vi "PH_ImageStatistician.panel.vi"(0 "object ref":refnum<vi>, 5 "error in (no error)":errorcluster) -> (19 "error out":errorcluster)   [LabVIEW 2014, in "PH_ImageStatistician.lvlib"]
doc: "This is just an example for a GUI thread.\n\nLicense Agreement for this software:\n\nCopyright (C)\nGesellschaft für Schwerionenforschung, GSI\nPlanckstr. 1\n64291 Darmstadt\nGermany\n\nContact: D.Beck@gsi.de \n\nThis program is free software; you can redistribute it and/or modify it under the terms of the GNU General Public License as published by the Free Software Foundation; either version 2 of the license, or (at your option) any later version.\n\nThis program is distributed in the hope that it will be useful, but WITHOUT ANYW ARRANTY; without even the implied warranty of MERCHANTABILITY or FITNESS FOR A PARTICULAR PURPOSE. See the GNU General License for more details (http://www.gnu.org).\n\nGesellschaft für Schwerionenforschung, GSI\nPlanckstr. 1, 64291 Darmstadt, Germany\nFor all questions and ideas contact: M.Richter@gsi.de, H.Brand@gsi.de or D.Beck@gsi.de.\nLast update: 18-DEC-2002"
uses:
  PH_ImageStatistician.lvlib
  PH_ImageStatistician.select Data.ctl
  PH_Common/PH_Common.lvlib
  CSCore/CSSystem/CSSystemLib/CSSystemLib.lvlib
  PH_Class/PH_Class.lvlib
panel:
  in  "Start":bool
  in  "Stat or Trend":bool
  in  "Export Data":bool
  out "Result Graph":cluster{dbl[], dbl[]}[](graph)
  out "Std Dev Data 3":dbl caption="Unit" format="%#_4g"
  in  "Dummy Std Dev":string caption="Std Dev"
  in  "Dummy Mean":string caption="Mean"
  out "Mean Data 3":dbl caption="Unit" format="%#_4g"
  out "Std Dev Data 2":dbl caption="Unit" format="%#_4g"
  out "Mean Data 2":dbl caption="Unit" format="%#_4g"
  out "Std Dev Data 1":dbl caption="Unit" format="%#_4g"
  out "Mean Data 1":dbl caption="Unit" format="%#_4g"
  in  "Data 3":T1 items=["nothing ", "FWHM Major Trace", "FWHM Minor Trace", "Gaussian Fit Order Major Trace", "Gaussian Fit Order Minor Trace", "99% Diameter Major Trace", "99% Diameter Minor Trace", "Theta", "Delta", "Major Diameter", "Minor Diameter", "Azimuth Angle", "Azi Angle rel to Major?", "Ellipticity", "Center of gravity - x", "Center of gravity - y", "Energy"]
  in  "Data 2":T1 items=["nothing ", "FWHM Major Trace", "FWHM Minor Trace", "Gaussian Fit Order Major Trace", "Gaussian Fit Order Minor Trace", "99% Diameter Major Trace", "99% Diameter Minor Trace", "Theta", "Delta", "Major Diameter", "Minor Diameter", "Azimuth Angle", "Azi Angle rel to Major?", "Ellipticity", "Center of gravity - x", "Center of gravity - y", "Energy"]
  in  "Data 1":T1 items=["nothing ", "FWHM Major Trace", "FWHM Minor Trace", "Gaussian Fit Order Major Trace", "Gaussian Fit Order Minor Trace", "99% Diameter Major Trace", "99% Diameter Minor Trace", "Theta", "Delta", "Major Diameter", "Minor Diameter", "Azimuth Angle", "Azi Angle rel to Major?", "Ellipticity", "Center of gravity - x", "Center of gravity - y", "Energy"]
  out "Status":u32(colorbox)
  in  "Operator":string
  in  "Delete":bool
  # "PCS"
  # "3.40"
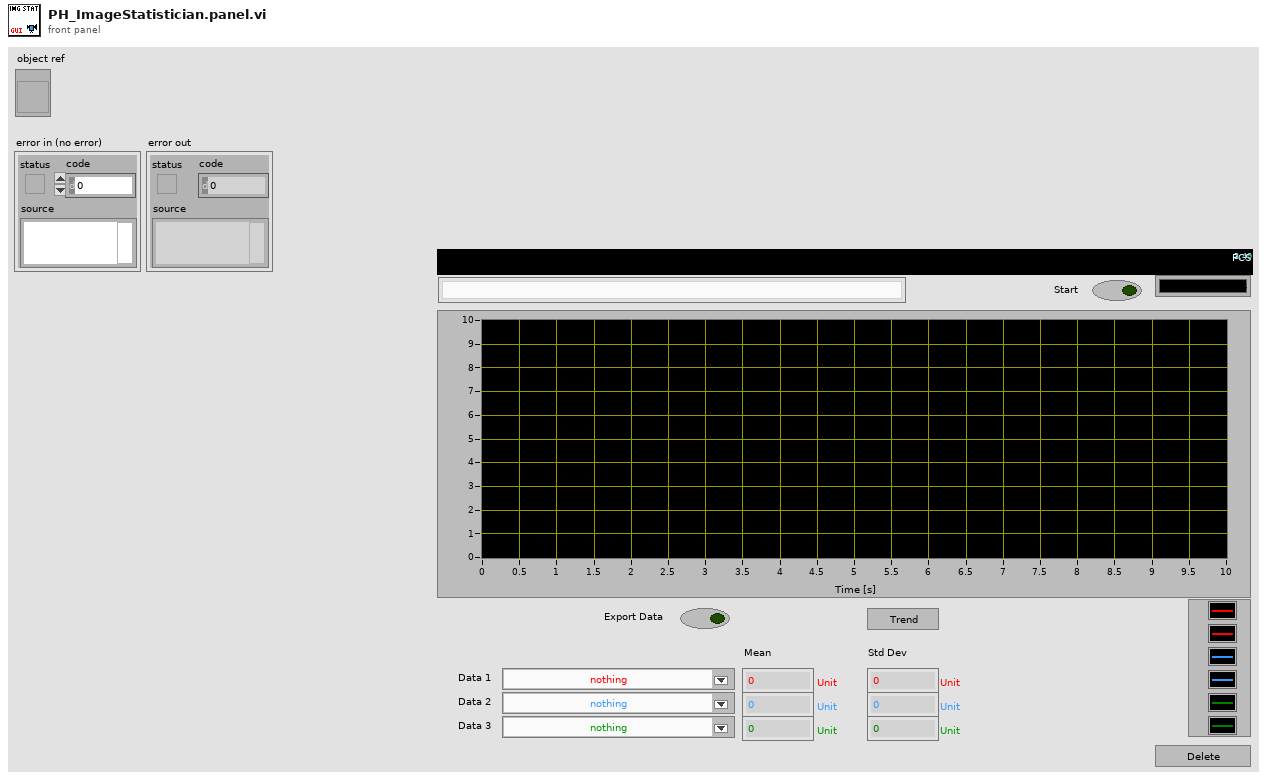
[diagram p1: front panel]
types:
  T1 = typedef "PH_ImageStatistician.lvlib/PH_ImageStatistician.select Data.ctl" = u16
  T2 = enum8{"Enabled", "Disabled", "Disabled and Grayed Out"}
  T3 = typedef "PH_ImageStatistician.lvlib/PH_ImageStatistician.i attribute.ctl" = cluster{"GUI Refs ":cluster{"Status":refnum<vi>, "Result Graph":refnum<vi>, "Mean Data 1":refnum<vi>, "Std Dev Data 1":refnum<vi>, "Mean Data 2":refnum<vi>, "Std Dev Data 2":refnum<vi>, "Mean Data 3":refnum<vi>, "Std Dev Data 3":refnum<vi>, "Dummy Mean":refnum<vi>, "Dummy Std Dev":refnum<vi>, "Export Data":refnum<vi>, "Data 1":refnum<vi>, "Data 2":refnum<vi>, "Data 3":refnum<vi>, "Stat or Trend":refnum<vi>, "Delete":refnum<vi>, "Operator":refnum<vi>, "Start":refnum<vi>}, "Operator":string, "Data":T4[], "Stat or Trend":bool, "Data 1":T1, "Data 2":T1, "Data 3":T1, "Start":bool, "Datasets strored":i32, "Dataarray Size":i32}
  T4 = typedef "PH_ImageStatistician.lvlib/PH_ImageStatistician.Statistician Data.ctl" = cluster{"Snapshot Time":dbl, "Maj FWHM":dbl, "Min FWHM":dbl, "Maj Fit Order":dbl, "Min Fit Order":dbl, "99% Diam Maj Trace":dbl, "99% Diam Min Trace":dbl, "Theta":dbl, "Delta":dbl, "Maj Diam":dbl, "Min Diam":dbl, "Azimuth Angle":dbl, "Azi Angle rel to major?":dbl, "Ellipticity":dbl, "CoG - X":dbl, "CoG - Y":dbl, "Energy":dbl, "Energy Cal - no mJ":dbl, "Lin Cal - no mm or mrad":dbl, "Lin Cal Factor":dbl}
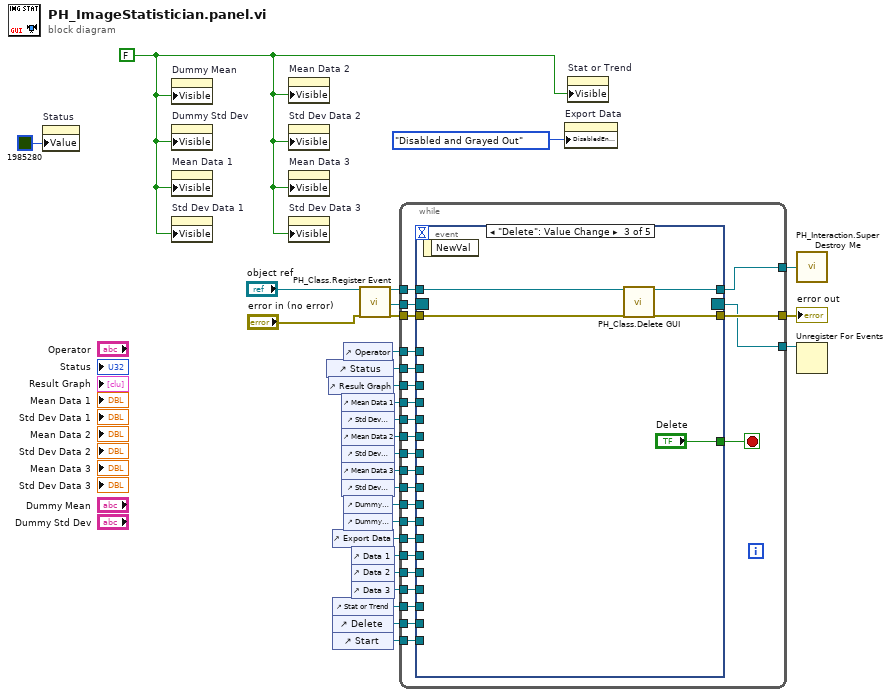
[diagram p0: block diagram]
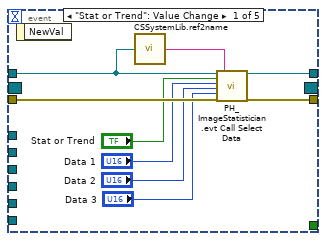
[diagram p2: hidden frame]
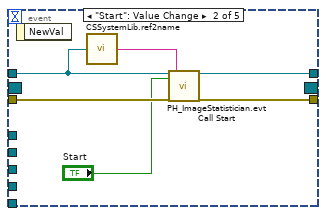
[diagram p3: hidden frame]
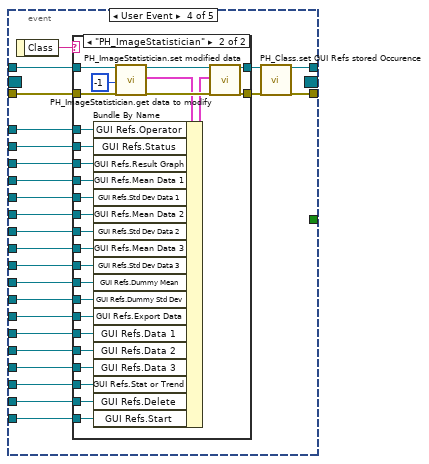
[diagram p4: hidden frame]
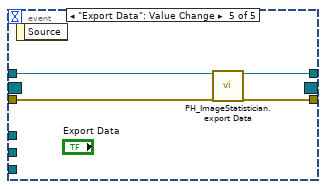
[diagram p6: hidden frame]
diagram:
  w27 = FALSE
  n1 = property on="Status" class="ColBox"("Value"=u32 1985280 ("Status")) -> ()  [unwired: 2 in, 2 out]
  n2 = property on="Dummy Mean" class="Str"("Visible"=w27) -> ()  [unwired: 2 in, 2 out]
  n3 = property on="Dummy Std Dev" class="Str"("Visible"=w27) -> ()  [unwired: 2 in, 2 out]
  n4 = property on="Mean Data 1" class="DigNum (strict)"("Visible"=w27) -> ()  [unwired: 2 in, 2 out]
  n5 = property on="Std Dev Data 1" class="DigNum (strict)"("Visible"=w27) -> ()  [unwired: 2 in, 2 out]
  n6 = property on="Mean Data 2" class="DigNum (strict)"("Visible"=w27) -> ()  [unwired: 2 in, 2 out]
  n7 = property on="Std Dev Data 2" class="DigNum (strict)"("Visible"=w27) -> ()  [unwired: 2 in, 2 out]
  n8 = property on="Mean Data 3" class="DigNum (strict)"("Visible"=w27) -> ()  [unwired: 2 in, 2 out]
  n9 = property on="Std Dev Data 3" class="DigNum (strict)"("Visible"=w27) -> ()  [unwired: 2 in, 2 out]
  n10 = control-ref of="Status"() -> (w17:refnum<vi>)
  n11 = control-ref of="Result Graph"() -> (w16:refnum<vi>)
  n12 = control-ref of="Export Data"() -> (w7:refnum<vi>)
  n13 = control-ref of="Stat or Trend"() -> (w3:refnum<vi>)
  n14 = control-ref of="Delete"() -> (w2:refnum<vi>)
  n15 = control-ref of="Start"() -> (w1:refnum<vi>)
  n16 = control-ref of="Mean Data 1"() -> (w15:refnum<vi>)
  n17 = control-ref of="Std Dev Data 1"() -> (w14:refnum<vi>)
  n18 = control-ref of="Mean Data 2"() -> (w13:refnum<vi>)
  n19 = control-ref of="Std Dev Data 2"() -> (w12:refnum<vi>)
  n20 = control-ref of="Mean Data 3"() -> (w11:refnum<vi>)
  n21 = control-ref of="Std Dev Data 3"() -> (w10:refnum<vi>)
  n22 = control-ref of="Operator"() -> (w18:refnum<vi>)
  n23 = control-ref of="Dummy Mean"() -> (w9:refnum<vi>)
  n24 = control-ref of="Dummy Std Dev"() -> (w8:refnum<vi>)
  n25 = control-ref of="Data 1"() -> (w6:refnum<vi>)
  n26 = control-ref of="Data 2"() -> (w5:refnum<vi>)
  n27 = control-ref of="Data 3"() -> (w4:refnum<vi>)
  n28 = call "PH_Class.Register Event.vi"("i ref in"="object ref", "error in (no error)"="error in (no error)") -> ("i ref out"=w24:refnum<vi>, "Event Registration Refnum"=w22:refnum<event-registration>, "error out"=w23:errorcluster)  [unwired: 15 in]
  n29 = while {
    tunnel: w24 -> [w53]
    tunnel: [w52] -> w29
    tunnel: [w51] -> w28
    tunnel: w23 -> [w50]
    tunnel: w22 -> [w49]
    tunnel: [w48] -> w21
    tunnel: w18 -> [w47]
    tunnel: w17 -> [w46]
    tunnel: w16 -> [w45]
    tunnel: w15 -> [w44]
    tunnel: w14 -> [w43]
    tunnel: w13 -> [w42]
    tunnel: w12 -> [w41]
    tunnel: w11 -> [w40]
    tunnel: w10 -> [w39]
    tunnel: w9 -> [w38]
    tunnel: w8 -> [w37]
    tunnel: w7 -> [w36]
    tunnel: w6 -> [w35]
    tunnel: w5 -> [w34]
    tunnel: w4 -> [w33]
    tunnel: w3 -> [w32]
    tunnel: w2 -> [w31]
    tunnel: w1 -> [w30]
    stop <- w54 stop-if-true
    n30 = event shown="[2] \"Delete\": Value Change" {
      selector: w49 -> [_ _ _ _ _]
      dyn-events: [_ _ _ _ _] -> w48
      timeout: _ -> [_ _ _ _ _]
      tunnel: [_ _ "Delete" _ _] -> w54
      tunnel: w53 -> [w59 w65 w73 w99 w131]
      tunnel: [w61 w67 w72 w95 w129] -> w52
      tunnel: [w62 w68 w70 w94 w130] -> w51
      tunnel: w50 -> [w63 w69 w71 w98 w132]
      tunnel: w47 -> [_ _ _ w92 _]
      tunnel: w46 -> [_ _ _ w91 _]
      tunnel: w45 -> [_ _ _ w90 _]
      tunnel: w44 -> [_ _ _ w89 _]
      tunnel: w43 -> [_ _ _ w88 _]
      tunnel: w42 -> [_ _ _ w87 _]
      tunnel: w41 -> [_ _ _ w86 _]
      tunnel: w40 -> [_ _ _ w85 _]
      tunnel: w39 -> [_ _ _ w84 _]
      tunnel: w38 -> [_ _ _ w83 _]
      tunnel: w37 -> [_ _ _ w82 _]
      tunnel: w36 -> [_ _ _ w81 _]
      tunnel: w35 -> [_ _ _ w80 _]
      tunnel: w34 -> [_ _ _ w79 _]
      tunnel: w33 -> [_ _ _ w78 _]
      tunnel: w32 -> [_ _ _ w77 _]
      tunnel: w31 -> [_ _ _ w76 _]
      tunnel: w30 -> [_ _ _ w75 _]
      event "Stat or Trend": Value Change {
        n31 = event-data() -> ()  [unwired: 1 in, 1 out]
        n32 = call "CSSystemLib.ref2name.vi"("obj refnum"=w59) -> ("name"=w60:string)
        n33 = call "PH_ImageStatistician.evt Call Select Data.vi"("i ref in"=w59, "Stat or Trend"="Stat or Trend", "Data 1"="Data 1", "Data 2"="Data 2", "Data 3"="Data 3", "error in (no error)"=w63, "Instance"=w60) -> ("i ref out"=w61:refnum<vi>, "error out"=w62:errorcluster)  [unwired: 11 in]
      }
      event "Start": Value Change {
        n34 = event-data() -> ()  [unwired: 1 in, 1 out]
        n35 = call "CSSystemLib.ref2name.vi"("obj refnum"=w65) -> ("name"=w66:string)
        n36 = call "PH_ImageStatistician.evt Call Start.vi"("i ref in"=w65, "Start"="Start", "error in (no error)"=w69, "Instance"=w66) -> ("i ref out"=w67:refnum<vi>, "error out"=w68:errorcluster)  [unwired: 14 in]
      }
      event "Delete": Value Change {
        n37 = event-data() -> ()  [unwired: 1 in, 1 out]
        n38 = call "PH_Class.Delete GUI.vi"("VI in"=w73, "error in (no error)"=w71) -> ("VI out"=w72:refnum<vi>, "error out"=w70:errorcluster)  [unwired: 16 in]
      }
      event User Event {
        n39 = event-data() -> ("Class"=w93:string)  [unwired: 1 in]
        n40 = case shown="\"PH_ImageStatistician\"" w93 {
          tunnel: w99 -> [w101 w123]
          tunnel: w98 -> [w100 w122]
          tunnel: [w100 w121] -> w97
          tunnel: [w101 w120] -> w96
          tunnel: w92 -> [_ w119]
          tunnel: w91 -> [_ w118]
          tunnel: w90 -> [_ w117]
          tunnel: w89 -> [_ w116]
          tunnel: w88 -> [_ w115]
          tunnel: w87 -> [_ w114]
          tunnel: w86 -> [_ w113]
          tunnel: w85 -> [_ w112]
          tunnel: w84 -> [_ w111]
          tunnel: w83 -> [_ w110]
          tunnel: w82 -> [_ w109]
          tunnel: w81 -> [_ w108]
          tunnel: w80 -> [_ w107]
          tunnel: w79 -> [_ w106]
          tunnel: w78 -> [_ w105]
          tunnel: w77 -> [_ w104]
          tunnel: w76 -> [_ w103]
          tunnel: w75 -> [_ w102]
          frame Default {
          }
          frame "PH_ImageStatistician" {
            n41 = call "PH_ImageStatistician.get data to modify.vi"("i ref in"=w123, "ms timeout (10000)"=-1, "error in (no error)"=w122) -> ("i ref out"=w127:refnum<vi>, "i attribute"=w125:T3, "error out"=w128:errorcluster)  [unwired: 13 in, 1 out]
            n42 = Bundle By Name(cluster=w125, "GUI Refs.Operator"=w119, "GUI Refs.Status"=w118, "GUI Refs.Result Graph"=w117, "GUI Refs.Mean Data 1"=w116, "GUI Refs.Std Dev Data 1"=w115, "GUI Refs.Mean Data 2"=w114, "GUI Refs.Std Dev Data 2"=w113, "GUI Refs.Mean Data 3"=w112, "GUI Refs.Std Dev Data 3"=w111, "GUI Refs.Dummy Mean"=w110, "GUI Refs.Dummy Std Dev"=w109, "GUI Refs.Export Data"=w108, "GUI Refs.Data 1"=w107, "GUI Refs.Data 2"=w106, "GUI Refs.Data 3"=w105, "GUI Refs.Stat or Trend"=w104, "GUI Refs.Delete"=w103, "GUI Refs.Start"=w102) -> (w124:T3)
            n43 = call "PH_ImageStatistician.set modified data.vi"("i ref in"=w127, "i attribute"=w124, "error in (no error)"=w128) -> ("i ref out"=w120:refnum<vi>, "error out"=w121:errorcluster)  [unwired: 15 in]
          }
        }
        n44 = call "PH_Class.set GUI Refs stored Occurence.vi"("i ref in"=w96, "error in (no error)"=w97) -> ("i ref out"=w95:refnum<vi>, "error out"=w94:errorcluster)  [unwired: 16 in]
      }
      event "Export Data": Value Change {
        n45 = event-data() -> ()  [unwired: 1 in, 1 out]
        n46 = call "PH_ImageStatistician.export Data.vi"("i ref in"=w131, "error in (no error)"=w132) -> ("i ref out"=w129:refnum<vi>, "error out"=w130:errorcluster)  [unwired: 16 in]
      }
    }
  }
  "error out" <- w28
  n47 = property on="Export Data" class="Bool"("DisabledEnum"=T2."Disabled and Grayed Out" ("Disabled")) -> ()  [unwired: 2 in, 2 out]
  n48 = property on="Stat or Trend" class="Bool (strict)"("Visible"=w27) -> ()  [unwired: 2 in, 2 out]
  n49 = call "PH_Interaction.Super Destroy Me.vi"("i ref out"=w29) -> ()
  n50 = Unregister For Events(event registration refnum=w21) -> ()  [unwired: 1 in, 1 out]
